vi "initialisation.vi"(11 "Queues in":T1) -> ()   [LabVIEW 2018]
uses:
  type defs/Queues.ctl
  <vilib>/LabVIEW Targets/FPGA/cRIO/shared/nicrio_ModuleControls/nicrio_cRIO-9237_DataRatesRing.ctl
  supporting VIs/polymorphic VIs/enqueue for comms.vi
  supporting VIs/polymorphic VIs/enqueue for data processor.vi
  supporting VIs/polymorphic VIs/enqueue for file IO.vi
  supporting VIs/polymorphic VIs/enqueue for data stream.vi
  supporting VIs/polymorphic VIs/enqueue for message handler.vi
  supporting VIs/polymorphic VIs/enqueue for user interface.vi
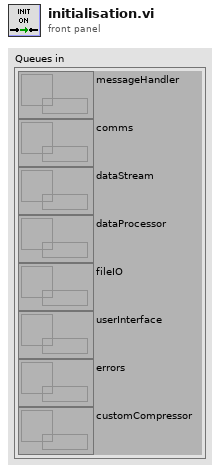
[diagram p1: front panel]
types:
  T1 = typedef "Queues.ctl" = cluster{"messageHandler":refnum<queue>, "comms":refnum<queue>, "dataStream":refnum<queue>, "dataProcessor":refnum<queue>, "fileIO":refnum<queue>, "userInterface":refnum<queue>, "errors":refnum<queue>, "customCompressor":refnum<queue>}
  T2 = typedef "nicrio_cRIO-9237_DataRatesRing.ctl" = u8
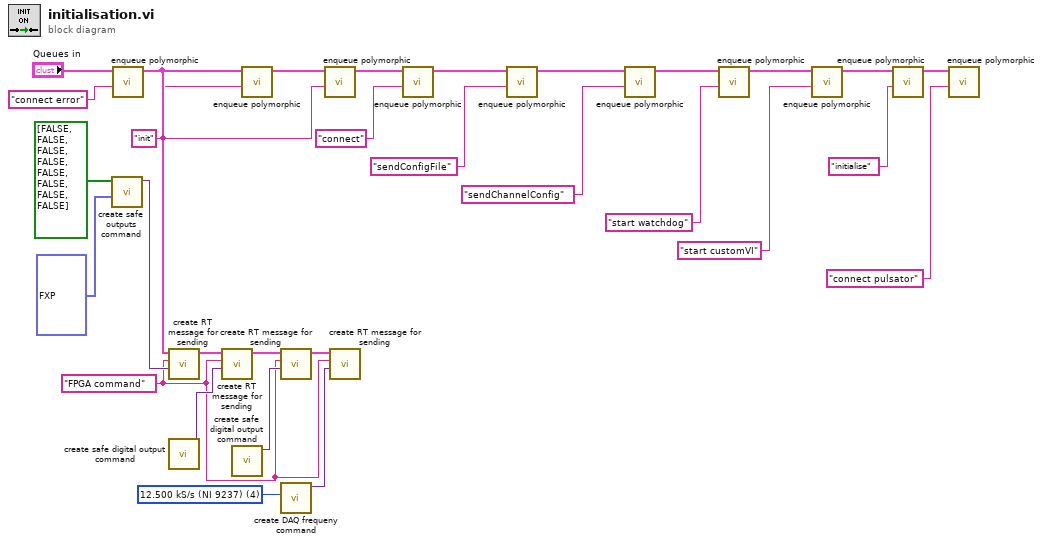
[diagram p0: block diagram]
diagram:
  w3 = T2 4 items=["50.000 kS/s (NI 9237)"=1, "25.000 kS/s (NI 9237)"=2, "16.667 kS/s (NI 9237)"=3, "12.500 kS/s (NI 9237)"=4, "10.000 kS/s (NI 9237)"=5, "8.333 kS/s (NI 9237)"=6, "7.143 kS/s (NI 9237)"=7, "6.250 kS/s (NI 9237)"=8, "5.556 kS/s (NI 9237)"=9, "5.000 kS/s (NI 9237)"=10, "4.545 kS/s (NI 9237)"=11, "4.167 kS/s (NI 9237)"=12, "3.846 kS/s (NI 9237)"=13, "3.571 kS/s (NI 9237)"=14, "3.333 kS/s (NI 9237)"=15, "3.125 kS/s (NI 9237)"=16, "2.941 kS/s (NI 9237)"=17, "2.778 kS/s (NI 9237)"=18, "2.632 kS/s (NI 9237)"=19, "2.500 kS/s (NI 9237)"=20, "2.381 kS/s (NI 9237)"=21, "2.273 kS/s (NI 9237)"=22, "2.174 kS/s (NI 9237)"=23, "2.083 kS/s (NI 9237)"=24, "2.000 kS/s (NI 9237)"=25, "1.923 kS/s (NI 9237)"=26, "1.852 kS/s (NI 9237)"=27, "1.786 kS/s (NI 9237)"=28, "1.724 kS/s (NI 9237)"=29, "1.667 kS/s (NI 9237)"=30, "1.613 kS/s (NI 9237)"=31] ("Data Rate")
  w1 = "FPGA command"
  w5 = "init" ("message")
  n1 = call "create safe outputs command.vi"("Safe Voltage"=fxp<+/-,20,5>[] [0.0, 0.0, 0.0, 0.0], "Safe Digital"=bool[] [FALSE, FALSE, FALSE, FALSE, FALSE, FALSE, FALSE, FALSE]) -> ("command message"=w18:variant)  [unwired: 9 in]
  n2 = call-poly "enqueue polymorphic.vi"("message"="connect error", "Queues"="Queues in") -> ("Queues out"=w19:T1)  [unwired: 9 in]
  n3 = call "create RT message for sending.vi"("RT data"=w18, "RT message"=w1, "Queues in"=w19) -> ("Queues out"=w15:T1)  [unwired: 8 in]
  n4 = call "create safe digital output command.vi"() -> ("command message"=w13:variant)  [unwired: 11 in]
  n5 = call "create RT message for sending.vi"("RT data"=w13, "RT message"=w1, "Queues in"=w15) -> ("Queues out"=w14:T1)  [unwired: 8 in]
  n6 = call "create safe digital output command.vi"() -> ("command message"=w12:variant)  [unwired: 11 in]
  n7 = call-poly "enqueue polymorphic.vi"("message"=w5, "Queues"=w19) -> ("Queues out"=w7:T1)  [unwired: 9 in]
  n8 = call "create RT message for sending.vi"("RT data"=w12, "RT message"=w1, "Queues in"=w14) -> ("Queues out"=w2:T1)  [unwired: 8 in]
  n9 = call "create DAQ frequeny command.vi"("Data Rate"=w3) -> ("command message"=w4:variant)  [unwired: 10 in]
  n10 = call-poly "enqueue polymorphic.vi"("message"=w5, "Queues"=w7) -> ("Queues out"=w6:T1)  [unwired: 9 in]
  n11 = call "create RT message for sending.vi"("RT data"=w4, "RT message"=w1, "Queues in"=w2) -> ()  [unwired: 8 in, 1 out]
  n12 = call-poly "enqueue polymorphic.vi"("message"="connect", "Queues"=w6) -> ("Queues out"=w27:T1)  [unwired: 9 in]
  n13 = call-poly "enqueue polymorphic.vi"("message"="sendConfigFile", "Queues"=w27) -> ("Queues out"=w25:T1)  [unwired: 9 in]
  n14 = call-poly "enqueue polymorphic.vi"("message"="sendChannelConfig", "Queues"=w25) -> ("Queues out"=w23:T1)  [unwired: 9 in]
  n15 = call-poly "enqueue polymorphic.vi"("message"="start watchdog", "Queues"=w23) -> ("Queues out"=w21:T1)  [unwired: 9 in]
  n16 = call-poly "enqueue polymorphic.vi"("message"="start customVI", "Queues"=w21) -> ("Queues out"=w11:T1)  [unwired: 9 in]
  n17 = call-poly "enqueue polymorphic.vi"("message"="initialise", "Queues"=w11) -> ("Queues out"=w9:T1)  [unwired: 9 in]
  n18 = call-poly "enqueue polymorphic.vi"("message"="connect pulsator", "Queues"=w9) -> ()  [unwired: 9 in, 1 out]
